vi "read_position.vi"(11 "Bytes in":refnum<class "Bytes.lvclass">) -> (2 "position":i32)   [LabVIEW 2020, in "Bytes.lvclass"]
uses:
  Bytes.lvclass
  Bytes.lvclass/Bytes.ctl
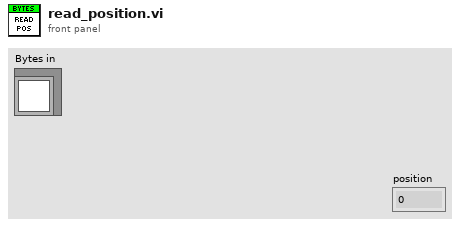
[diagram p1: front panel]
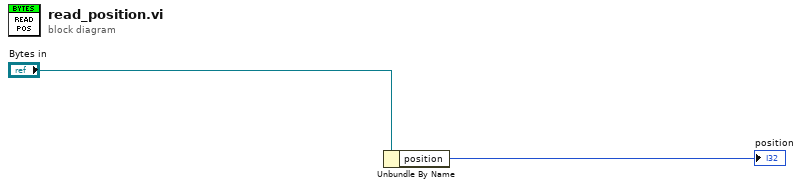
[diagram p0: block diagram]
diagram:
  n1 = Unbundle By Name("Bytes in") -> ("position"=→"position":i32)
